vi "play song.vi"   [LabVIEW 2023]
uses:
  <vilib>/sound2/lvsound2.llb/Sampling Mode.ctl
  <vilib>/sound2/lvsound2.llb/Sound File Info (path).vi
  <vilib>/sound2/lvsound2.llb/Sound File Read Open.vi
  <vilib>/sound2/lvsound2.llb/Sound File Read (DBL).vi
  <vilib>/sound2/lvsound2.llb/Sound Output Write (DBL).vi
types:
  T1 = typedef "Sampling Mode.ctl" = i32
  T2 = typedef "Sound Data Format.ctl" = cluster{"sample rate (S/s)":dbl, "number of channels":i32, "bits per sample":i32}
  T3 = typedef "Sound File Refnum.ctl" = refnum<file>
  T4 = typedef "Sound Output Task ID.ctl" = u32
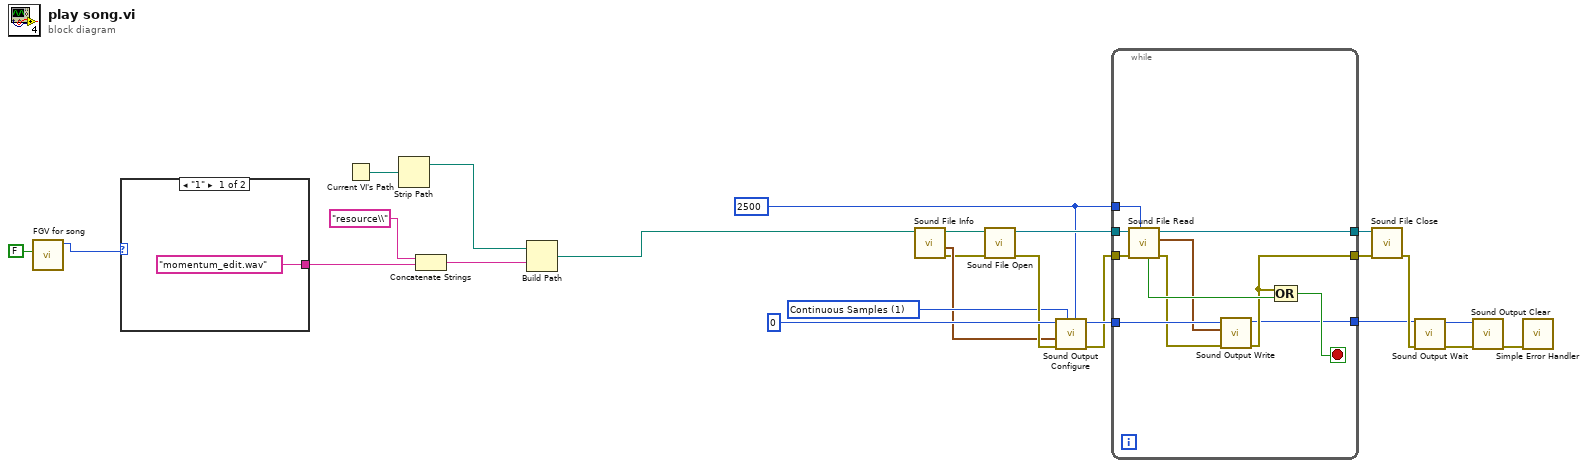
[diagram p0: block diagram]
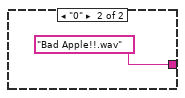
[diagram p2: hidden frame]
diagram:
  w16 = 2500 ("number of samples/ch")
  w12 = T1 1 items=["Finite Samples", "Continuous Samples"] ("sample mode")
  n1 = call "FGV for song.vi"("mode"=FALSE) -> ("read song"=w7:enum16{"0", "1"})  [unwired: 10 in]
  n2 = case shown="\"1\"" w7 {
    tunnel: ["momentum_edit.wav" ("string") "Bad Apple!!.wav" ("string")] -> w3
    frame "1" {
    }
    frame "0" {
    }
  }
  n3 = Current VI's Path() -> (path=w6:path)
  n4 = Strip Path(path=w6) -> (stripped path=w5:path)  [unwired: 1 out]
  n5 = Concatenate Strings("resource\\" ("string"), w3) -> (w2:string)
  n6 = Build Path(base path=w5, name or relative path=w2) -> (appended path=w4:path)
  n7 = call-poly <vilib>:"Sound File Info.vi"("path"=w4) -> ("error out"=w10:errorcluster, "sound format"=w11:T2, "path out"=w9:path)  [unwired: 7 in, 1 out]
  n8 = call-poly <vilib>:"Sound File Open.vi"("error in (no error)"=w10, "path"=w9) -> ("error out"=w13:errorcluster, "sound file refnum"=w17:T3)  [unwired: 8 in]
  n9 = call <vilib>:"Sound Output Configure.vi"("number of samples/ch"=w16, "sample mode"=w12, "error in (no error)"=w13, "sound format"=w11, "device ID"=u32 0) -> ("error out"=w15:errorcluster, "task ID"=w18:T4)  [unwired: 5 in]
  n10 = while {
    tunnel: w15 -> [w38]
    tunnel: w16 -> [w37]
    tunnel: w17 -> [w36]
    tunnel: [w33] -> w19
    tunnel: w18 -> [w32]
    tunnel: [w29] -> w20
    tunnel: [w28] -> w21
    stop <- w34 stop-if-true
    n11 = call-poly <vilib>:"Sound File Read.vi"("number of samples/ch (-1: all)"=w37, "error in (no error)"=w38, "sound file refnum"=w36) -> ("error out"=w31:errorcluster, "data"=w30:waveform(dbl)[], "sound file refnum out"=w33:T3, "end of file?"=w35:bool)  [unwired: 4 in, 1 out]
    n12 = call-poly <vilib>:"Sound Output Write.vi"("error in (no error)"=w31, "data"=w30, "task ID"=w32) -> ("error out"=w29:errorcluster, "task ID out"=w28:T4)  [unwired: 7 in]
    n13 = Compound Arithmetic op=OR(w29, w35) -> (w34:bool)
  }
  n14 = call <vilib>:"Sound File Close.vi"("error in (no error)"=w20, "sound file refnum"=w19) -> ("error out"=w22:errorcluster)  [unwired: 9 in]
  n15 = call <vilib>:"Sound Output Wait.vi"("error in (no error)"=w22, "task ID"=w21) -> ("error out"=w23:errorcluster, "task ID out"=w24:T4)  [unwired: 8 in]
  n16 = call <vilib>:"Sound Output Clear.vi"("error in (no error)"=w23, "task ID"=w24) -> ("error out"=w25:errorcluster)  [unwired: 9 in]
  n17 = call <vilib>:"Simple Error Handler.vi"("error in (no error)"=w25) -> ()  [unwired: 4 in, 5 out]
